vi "Write SQL Server.vi"(1 "connection information":string, 2 "error in (no error)":errorcluster, 3 "Data in":T1, 4 "table":string) -> (0 "error out":errorcluster)   [LabVIEW 2014]
uses:
  <vilib>/addons/database/Connection.llb/DB Tools Open Connec (String).vi
  <vilib>/addons/database/NI_Database_API.lvlib
panel:
  in  "?":string
  in  "?":string
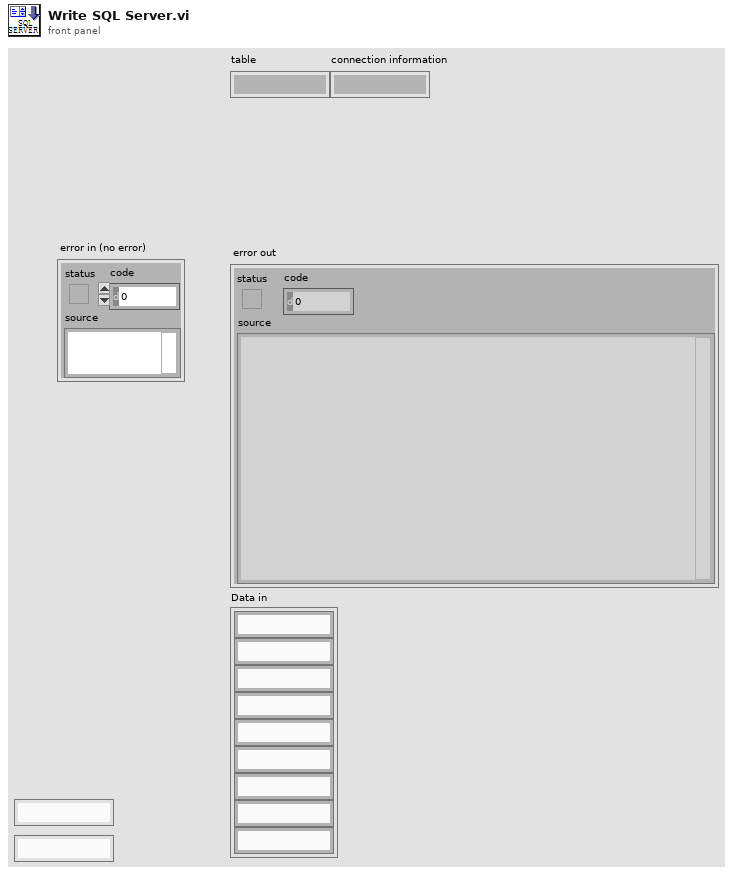
[diagram p1: front panel]
types:
  T1 = cluster{string, string, string, string, string, string, string, string, string}
  T2 = typedef "NI_Database_API.lvlib/Conn ObjectReference.ctl" = refnum<k1>
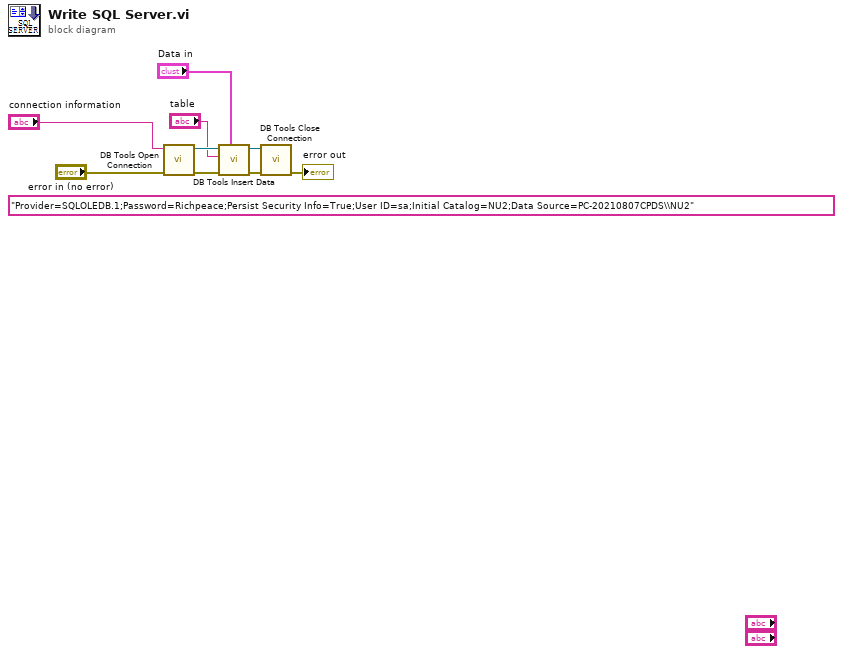
[diagram p0: block diagram]
diagram:
  (unwired) "Provider=SQLOLEDB.1;Password=Richpeace;Persist Security Info=True;User ID=sa;Initial Catalog=NU2;Data Source=PC-20210807CPDS\\NU2" ("table")
  n1 = call-poly <vilib>:"DB Tools Open Connection.vi"("error in (no error)"="error in (no error)", "connection information"="connection information") -> ("error out"=w8:errorcluster, "connection reference"=w9:T2)  [unwired: 6 in]
  n2 = call <vilib>:"DB Tools Insert Data.vi"("data"="Data in", "error in (no error)"=w8, "table"="table", "connection reference"=w9) -> ("error out"=w6:errorcluster, "connection reference out"=w5:T2)  [unwired: 6 in]
  n3 = call <vilib>:"DB Tools Close Connection.vi"("error in (no error)"=w6, "connection reference"=w5) -> ("error out"=→"error out":errorcluster)  [unwired: 5 in]
